vi "Add Attribute - Array.vi"(8 "error in (no error)":errorcluster, 9 "Value":refnum<class "YAML Parser.lvclass">, 10 "Attribute":string, 11 "YAML Parser in":refnum<class "YAML Parser.lvclass">) -> (0 "error out":errorcluster, 3 "YAML Parser out":refnum<class "YAML Parser.lvclass">)   [LabVIEW 2015, in "YAML Parser.lvclass"]
uses:
  YAML Parser.lvclass
panel:
  out "replaced":bool
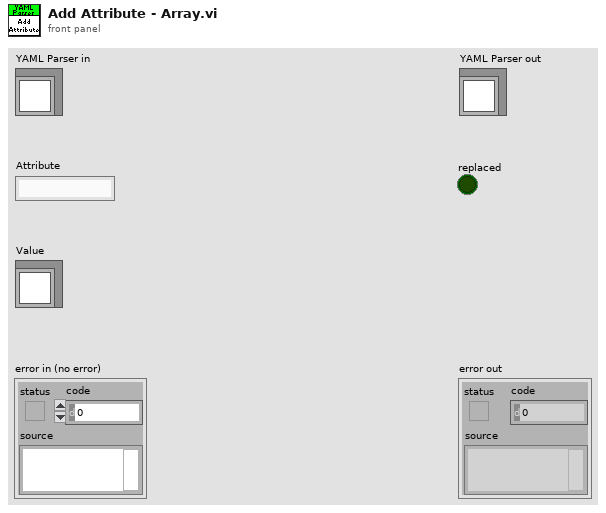
[diagram p1: front panel]
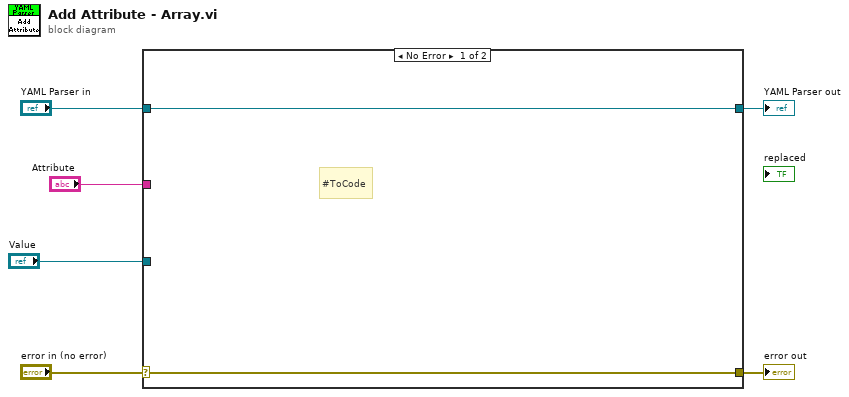
[diagram p0: block diagram]
diagram:
  n1 = case shown="No Error" "error in (no error)" {
    selector: "error in (no error)" -> [w7 w10]
    tunnel: [w7 w10] -> w5
    tunnel: [w8 w9] -> w3
    tunnel: "YAML Parser in" -> [w8 w9]
    tunnel: "Attribute" -> [_ _]
    tunnel: "Value" -> [_ _]
    frame No Error {
      # "#ToCode"
    }
    frame Error {
    }
  }
  "error out" <- w5
  "YAML Parser out" <- w3
